vi "readFromXML.vi"(8 "error in (no error)":errorcluster, 10 "XML in":string, 11 "SetOperatorAccessMode in":refnum<class "SetOperatorAccessMode.lvclass">) -> (0 "error out":errorcluster, 3 "SetOperatorAccessMode out":refnum<class "SetOperatorAccessMode.lvclass">)   [LabVIEW 2022 SP3, in "TCSDataDefinitions.lvlib" / "TCSCommand.lvlib" / "SetAccessMode.lvlib" / "SetOperatorAccessMode.lvclass"]
uses:
  SetOperatorAccessMode.lvclass
  SetAccessMode/SetAccessMode.lvclass
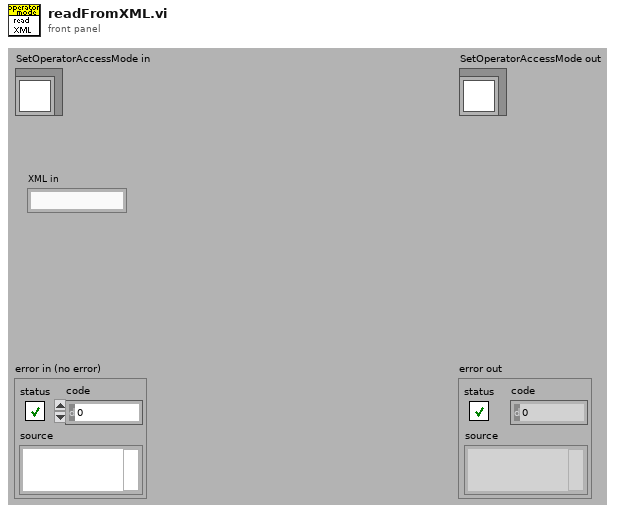
[diagram p1: front panel]
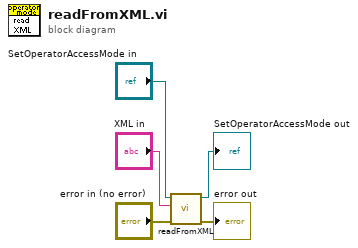
[diagram p0: block diagram]
diagram:
  n1 = call-parent "readFromXML.vi"("error in (no error)"="error in (no error)", "XML in"="XML in", "SetAccessMode in"="SetOperatorAccessMode in") -> ("error out"=→"error out":errorcluster, "SetAccessMode out"=→"SetOperatorAccessMode out":refnum<class "SetOperatorAccessMode.lvclass">)  [unwired: 7 out]
